vi "Terminal-Test-CheckAll.vi"(8 "error in (no error)":errorcluster caption="错误输入（无错误）", 11 "最大尝试次数":u32) -> (0 "error out":errorcluster caption="错误输出", 3 "布尔":bool)   [LabVIEW 2014]
uses:
  Terminal-Global-ReferenceValues.vi
  Terminal-Global-SetValues.vi
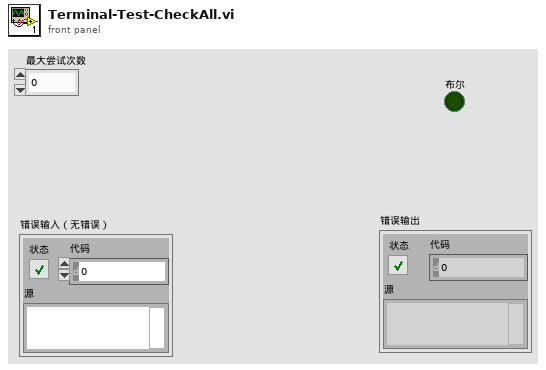
[diagram p1: front panel]
types:
  T1 = cluster{"径向油缸加载压力":u16, "轴向油缸加载压力":u16, "油箱1油液温度":u16, "润滑油温度":u16, "油箱2油液温度":u16, "试验轴承供油压力":u16, "试验轴承供油流量":u16, "陪试轴承供油流量":u16, "陪试轴承供油压力":u16, "陪试轴承供油温度":u16, "液压子系统状态字":cluster{"加载单元":cluster{"供油过滤器堵塞报警":bool, "回油过滤器堵塞报警":bool, "液位过高报警":bool, "液位过低报警":bool}, "试验轴承单元":cluster{"加热装置异常报警":bool, "油箱1液位过高报警":bool, "油箱1液位过低报警":bool, "油箱2液位过高报警":bool, "油箱2液位过低报警":bool, "供油过滤器堵塞报警":bool, "循环回路过滤器堵塞报警":bool, "回油过滤器堵塞报警":bool}, "陪试轴承单元":cluster{"供油过滤器1堵塞报警":bool, "供油过滤器2堵塞报警":bool, "回油过滤器堵塞报警":bool, "油箱液位过高报警":bool, "油箱液位过低报警":bool}}}
  T2 = cluster{"润滑油流量":u16, "油箱润滑油液位":u16, "油箱温度":u16, "冷却装置工作状态":u16, "供油压力":u16, "过滤器压差":u16, "油箱液位":u16, "供油油温":u16, "齿轮箱轴承温度":u16, "齿轮箱高速端输出转速":u16, "齿轮子系统状态字":cluster{"加热装置异常报警":bool, "冷却装置异常报警":bool, "油箱液位过低报警":bool, "供油油温过高报警":bool, "循环回路过滤器压差过高报警":bool, "1号油泵故障报警":bool, "2号油泵故障报警":bool, "供油压力过低报警":bool, "供油流量过低报警":bool, "轴承温度异常报警":bool, "油箱液位过高报警":bool, "回油过滤器压差过高报警":bool, "供油过滤器压差过高报警":bool}}
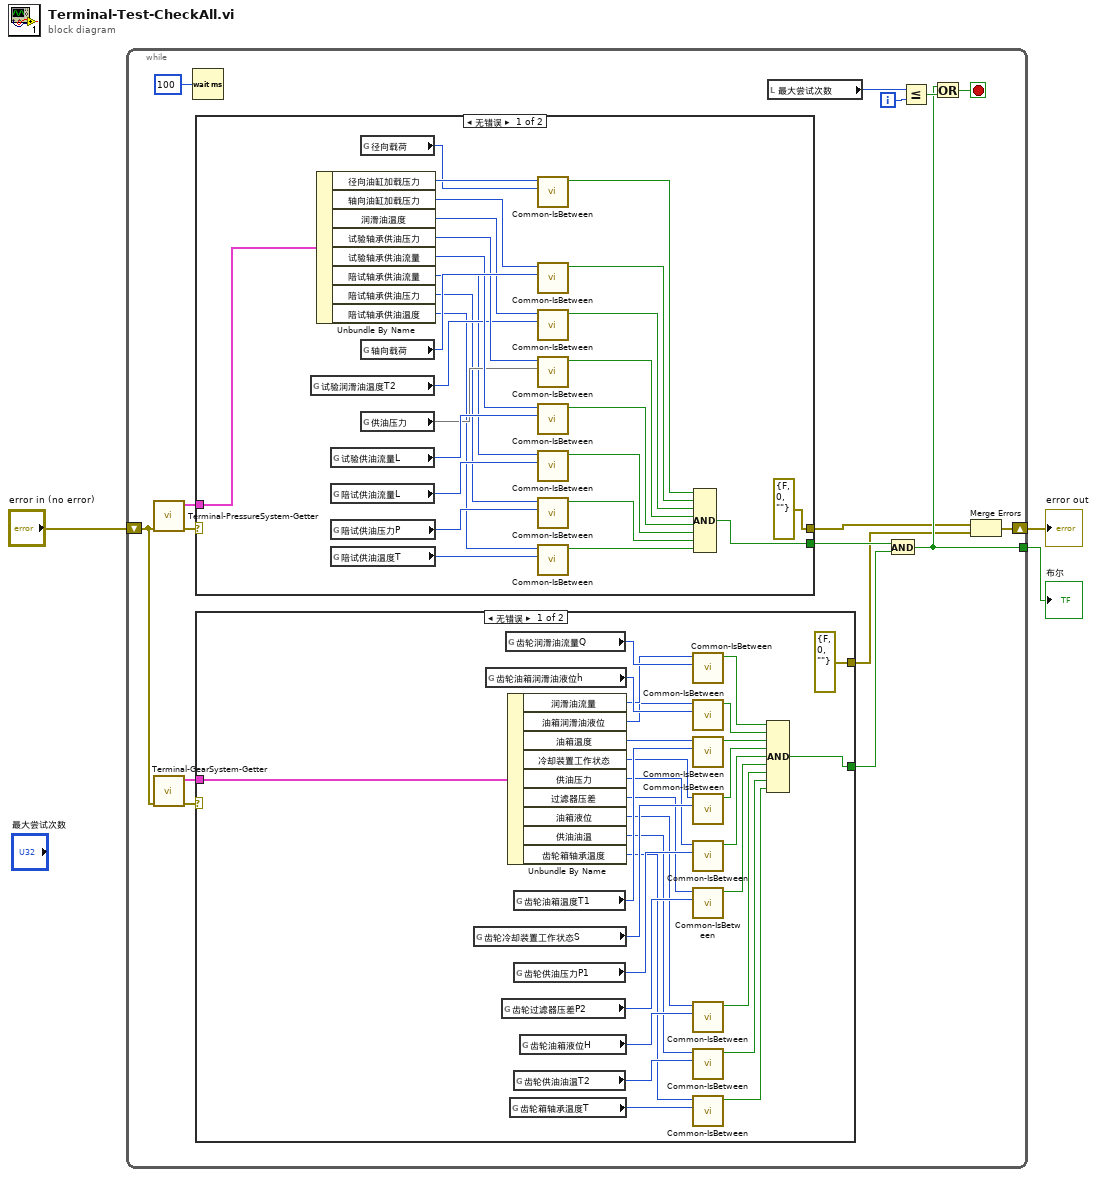
[diagram p0: block diagram]
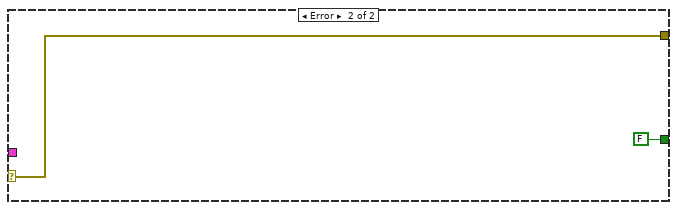
[diagram p2: hidden frame]
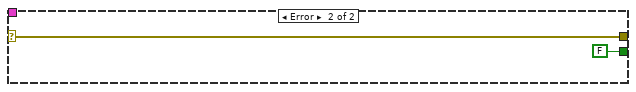
[diagram p3: hidden frame]
diagram:
  n1 = while {
    tunnel: [w8] -> w3
    shift-right: [w4] -> w1
    shift-left: "error in (no error)" -> [w7]
    i -> [w11]
    stop <- w9 stop-if-true
    n2 = call "Terminal-PressureSystem-Getter.vi"("error in (no error)"=w7) -> ("error out"=w19:errorcluster, "设备信息"=w18:T1)  [unwired: 9 in]
    n3 = call "Terminal-GearSystem-Getter.vi"("error in (no error)"=w7) -> ("error out"=w17:errorcluster, "设备信息"=w16:T2)  [unwired: 9 in]
    n4 = Wait (ms)(milliseconds to wait=u32 100 ("等待时间（毫秒）")) -> ()  [unwired: 1 out]
    n5 = case shown="无错误" w19 {
      selector: w19 -> [_ w79]
      tunnel: w18 -> [w78 _]
      tunnel: [w53 FALSE] -> w15
      tunnel: [errorcluster {"status"=FALSE, "code"=0, "source"=""} ("错误常量") w79] -> w5
      frame No Error {
        n6 = global read "Terminal-Global-ReferenceValues.vi" "试验润滑油温度T2"() -> (w63:u16)
        n7 = Unbundle By Name(w78) -> ("径向油缸加载压力"=w77:u16, "轴向油缸加载压力"=w74:u16, "润滑油温度"=w71:u16, "试验轴承供油压力"=w68:u16, "试验轴承供油流量"=w67:u16, "陪试轴承供油流量"=w59:u16, "陪试轴承供油压力"=w58:u16, "陪试轴承供油温度"=w57:u16)
        n8 = global read "Terminal-Global-ReferenceValues.vi" "试验供油流量L"() -> (w69:u16)
        n9 = global read "Terminal-Global-ReferenceValues.vi" "陪试供油流量L"() -> (w62:u16)
        n10 = global read "Terminal-Global-ReferenceValues.vi" "陪试供油压力P"() -> (w61:u16)
        n11 = global read "Terminal-Global-ReferenceValues.vi" "陪试供油温度T"() -> (w60:u16)
        n12 = global read "Terminal-Global-SetValues.vi" "径向载荷"() -> (w76:u16)
        n13 = global read "Terminal-Global-SetValues.vi" "轴向载荷"() -> (w75:u16)
        n14 = global read "Terminal-Global-SetValues.vi" "供油压力"() -> (w64)
        n15 = call "Common-IsBetween.vi"("基数"=w76, "x"=w77) -> ("范围内？"=w73:bool)  [unwired: 9 in]
        n16 = call "Common-IsBetween.vi"("基数"=w75, "x"=w74) -> ("范围内？"=w72:bool)  [unwired: 9 in]
        n17 = call "Common-IsBetween.vi"("基数"=w63, "x"=w71) -> ("范围内？"=w70:bool)  [unwired: 9 in]
        n18 = call "Common-IsBetween.vi"("基数"=w64, "x"=w68) -> ("范围内？"=w66:bool)  [unwired: 9 in]
        n19 = call "Common-IsBetween.vi"("基数"=w69, "x"=w67) -> ("范围内？"=w65:bool)  [unwired: 9 in]
        n20 = call "Common-IsBetween.vi"("基数"=w62, "x"=w59) -> ("范围内？"=w56:bool)  [unwired: 9 in]
        n21 = call "Common-IsBetween.vi"("基数"=w61, "x"=w58) -> ("范围内？"=w55:bool)  [unwired: 9 in]
        n22 = call "Common-IsBetween.vi"("基数"=w60, "x"=w57) -> ("范围内？"=w54:bool)  [unwired: 9 in]
        n23 = Compound Arithmetic op=AND(w73, w72, w70, w66, w65, w56, w55, w54) -> (w53:bool)
      }
      frame Error {
      }
    }
    n24 = case shown="无错误" w17 {
      selector: w17 -> [_ w50]
      tunnel: w16 -> [w49 _]
      tunnel: [w21 FALSE] -> w14
      tunnel: [errorcluster {"status"=FALSE, "code"=0, "source"=""} ("错误常量") w50] -> w6
      frame No Error {
        n25 = global read "Terminal-Global-ReferenceValues.vi" "齿轮冷却装置工作状态S"() -> (w45:u16)
        n26 = global read "Terminal-Global-ReferenceValues.vi" "齿轮油箱润滑油液位h"() -> (w47:u16)
        n27 = global read "Terminal-Global-ReferenceValues.vi" "齿轮过滤器压差P2"() -> (w42:u16)
        n28 = global read "Terminal-Global-ReferenceValues.vi" "齿轮润滑油流量Q"() -> (w48:u16)
        n29 = Unbundle By Name(w49) -> ("润滑油流量"=w39:u16, "油箱润滑油液位"=w38:u16, "油箱温度"=w37:u16, "冷却装置工作状态"=w36:u16, "供油压力"=w35:u16, "过滤器压差"=w34:u16, "油箱液位"=w33:u16, "供油油温"=w32:u16, "齿轮箱轴承温度"=w31:u16)
        n30 = global read "Terminal-Global-ReferenceValues.vi" "齿轮箱轴承温度T"() -> (w40:u16)
        n31 = global read "Terminal-Global-ReferenceValues.vi" "齿轮油箱温度T1"() -> (w46:u16)
        n32 = global read "Terminal-Global-ReferenceValues.vi" "齿轮供油压力P1"() -> (w41:u16)
        n33 = global read "Terminal-Global-ReferenceValues.vi" "齿轮供油油温T2"() -> (w44:u16)
        n34 = global read "Terminal-Global-ReferenceValues.vi" "齿轮油箱液位H"() -> (w43:u16)
        n35 = call "Common-IsBetween.vi"("基数"=w48, "x"=w39) -> ("范围内？"=w30:bool)  [unwired: 9 in]
        n36 = call "Common-IsBetween.vi"("基数"=w47, "x"=w38) -> ("范围内？"=w29:bool)  [unwired: 9 in]
        n37 = call "Common-IsBetween.vi"("基数"=w46, "x"=w37) -> ("范围内？"=w28:bool)  [unwired: 9 in]
        n38 = call "Common-IsBetween.vi"("基数"=w45, "x"=w36) -> ("范围内？"=w27:bool)  [unwired: 9 in]
        n39 = call "Common-IsBetween.vi"("基数"=w41, "x"=w35) -> ("范围内？"=w26:bool)  [unwired: 9 in]
        n40 = call "Common-IsBetween.vi"("基数"=w42, "x"=w34) -> ("范围内？"=w25:bool)  [unwired: 9 in]
        n41 = call "Common-IsBetween.vi"("基数"=w43, "x"=w33) -> ("范围内？"=w24:bool)  [unwired: 9 in]
        n42 = call "Common-IsBetween.vi"("基数"=w44, "x"=w32) -> ("范围内？"=w23:bool)  [unwired: 9 in]
        n43 = call "Common-IsBetween.vi"("基数"=w40, "x"=w31) -> ("范围内？"=w22:bool)  [unwired: 9 in]
        n44 = Compound Arithmetic op=AND(w30, w29, w28, w27, w26, w25, w24, w23, w22) -> (w21:bool)
      }
      frame Error {
      }
    }
    n45 = local read "最大尝试次数"() -> (w12:u32)
    n46 = And(x=w15, y=w14) -> (x .and. y?=w8:bool)
    n47 = Less Or Equal?(x=w12, y=w11) -> (x <= y?=w10:bool)
    n48 = Or(x=w8, y=w10) -> (x .or. y?=w9:bool)
    n49 = Merge Errors(w5, w6) -> (w4:errorcluster)
  }
  "布尔" <- w3
  "error out" <- w1
